vi "ma_Check Block Size (2ch) no State.vi"(0 "time signal X":waveform(dbl), 1 "averaging parameters":T3={"averaging mode"=enum."No averaging", "weighting mode"=enum."Exponential", "number of averages"=10} {"number of averages" min=1}, 5 "time signal Y":waveform(dbl), 9 "restart averaging (F)":bool, 11 "error in":errorcluster, 12 "caller VI name":string, 13 "state info":T1 {"Syy" format="%0.2f"; "Sxy" format="%0.2f"; "Sy" format="%0.2f"; "Sxx" format="%0.2f"; "avgs completed" format="%0.2f"; "df" format="%0.2f"; "Sx" format="%0.2f"; "spectrum parameters"."window" items=["Rectangle"=0, "Hanning"=1, "Hamming"=2, "Blackman-Harris"=3, "Exact Blackman"=4, "Blackman"=5, "Flat Top"=6, "4 Term B-Harris "=7, "7 Term B-Harris"=8, "Low Sidelobe"=9, "Blackman Nuttall"=11, "Triangle"=30, "Bartlett-Hanning"=31, "Bohman"=32, "Parzen"=33, "Welch"=34, "Kaiser"=60, "Dolph-Chebyshev"=61, "Gaussian"=62]; "dt" format="%0.2f"; "timestamp" format="%0.2f"; "dt history" format="%0.2f"; "t0 history" format="%0.2f"}) -> (4 "force restart averaging":bool, 14 "state info out":T1 {"Syy" format="%0.2f"; "Sxy" format="%0.2f"; "Sy" format="%0.2f"; "Sxx" format="%0.2f"; "avgs completed" format="%0.2f"; "df" format="%0.2f"; "Sx" format="%0.2f"; "spectrum parameters"."window" items=["Rectangle"=0, "Hanning"=1, "Hamming"=2, "Blackman-Harris"=3, "Exact Blackman"=4, "Blackman"=5, "Flat Top"=6, "4 Term B-Harris "=7, "7 Term B-Harris"=8, "Low Sidelobe"=9, "Blackman Nuttall"=11, "Triangle"=30, "Bartlett-Hanning"=31, "Bohman"=32, "Parzen"=33, "Welch"=34, "Kaiser"=60, "Dolph-Chebyshev"=61, "Gaussian"=62]; "dt" format="%0.2f"; "timestamp" format="%0.2f"; "dt history" format="%0.2f"; "t0 history" format="%0.2f"}, 15 "error out":errorcluster)   [LabVIEW 2020, in "NI_MAPro.lvlib"]
uses:
  NI_MAPro.lvlib
  2-chan State.ctl
  windowTd.ctl
  NI_MABase.lvlib
  NI_AALPro.lvlib
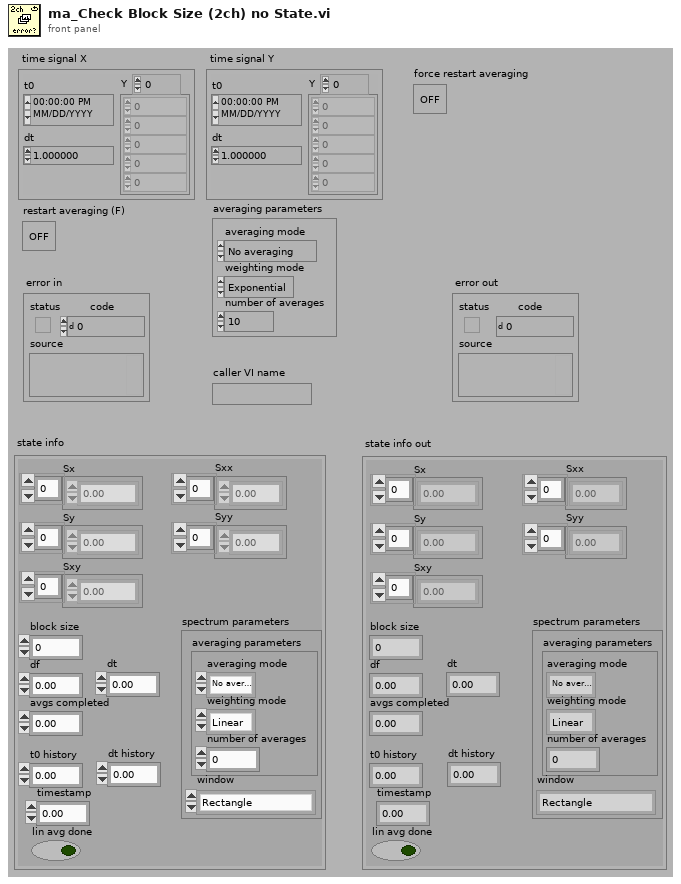
[diagram p1: front panel]
types:
  T1 = typedef "NI_MAPro.lvlib/2-chan State.ctl" = cluster{"Sx":cdb[], "Sy":cdb[], "Sxx":dbl[], "Syy":dbl[], "Sxy":cdb[], "block size":i32, "df":dbl, "dt":dbl, "avgs completed":dbl, "spectrum parameters":cluster{"averaging parameters":cluster{"averaging mode":enum16{"No averaging", "Vector averaging", "RMS averaging", "Peak hold"}, "weighting mode":enum16{"Linear", "Exponential"}, "number of averages":u32}, "window":T2}, "lin avg done":bool, "t0 history":dbl, "dt history":dbl, "timestamp":dbl}
  T2 = typedef "NI_AALPro.lvlib/windowTd.ctl" = u32
  T3 = cluster{"averaging mode":enum16{"No averaging", "Vector averaging", "RMS averaging", "Peak hold"}, "weighting mode":enum16{"Linear", "Exponential"}, "number of averages":u32}
  T4 = enum16{"No averaging", "Vector averaging", "RMS averaging", "Peak hold"}
  T5 = cluster{"status":bool, "code":i32, "caller VI name":string}
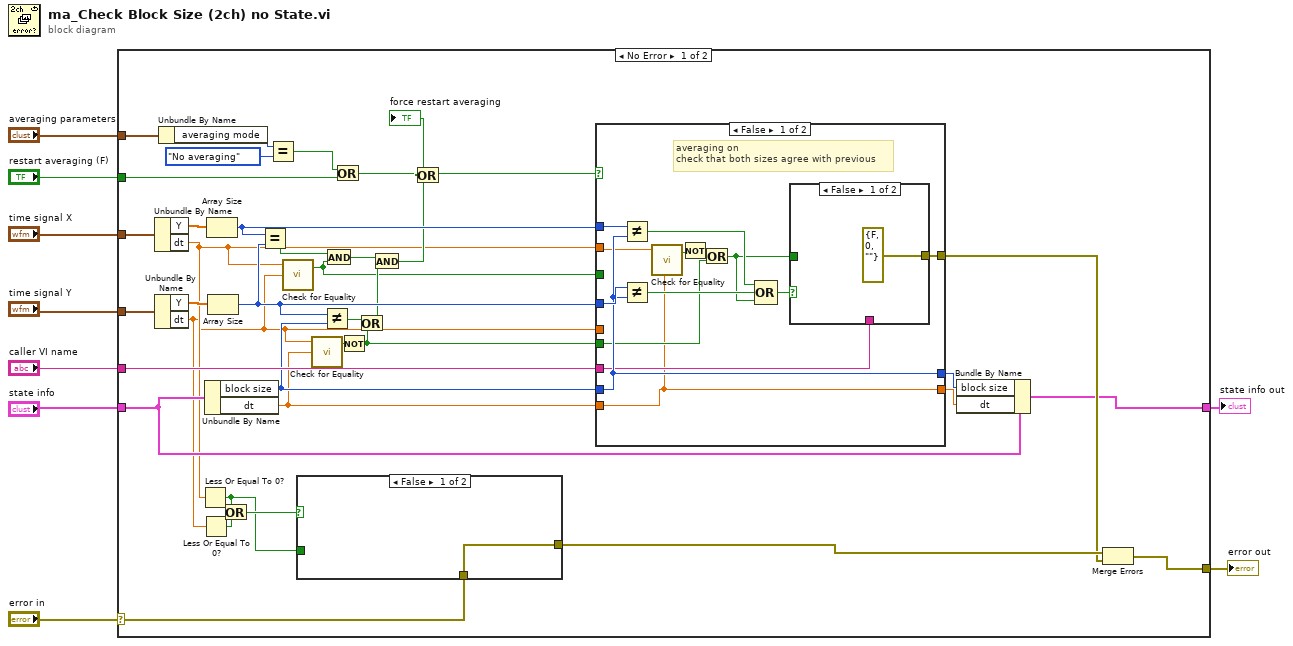
[diagram p0: block diagram]
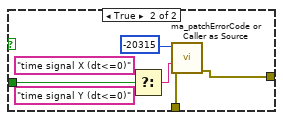
[diagram p2: hidden frame]
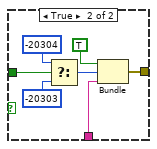
[diagram p3: hidden frame]
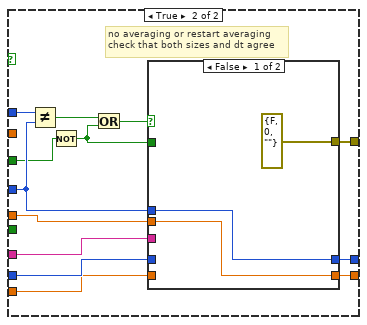
[diagram p4: hidden frame]
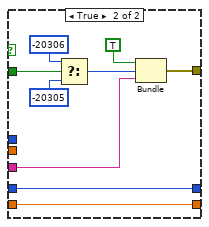
[diagram p5: hidden frame]
diagram:
  n1 = case shown="No Error" "error in" {
    selector: "error in" -> [w10 w103]
    tunnel: [w39 w103] -> w9
    tunnel: "time signal Y" -> [w46 _]
    tunnel: "time signal X" -> [w45 _]
    tunnel: "restart averaging (F)" -> [w44 _]
    tunnel: "averaging parameters" -> [w43 _]
    tunnel: "caller VI name" -> [w42 _]
    tunnel: "state info" -> [w38 w102]
    tunnel: [w17 w102] -> w1
    frame No Error {
      n2 = Unbundle By Name(w45) -> ("Y"=w37:dbl[], "dt"=w16:dbl)
      n3 = Unbundle By Name(w46) -> ("Y"=w36:dbl[], "dt"=w15:dbl)
      n4 = Unbundle By Name(w43) -> ("averaging mode"=w34:T4)
      n5 = Less Or Equal To 0?(x=w16) -> (x <= 0?=w21:bool)
      n6 = Less Or Equal To 0?(x=w15) -> (x <= 0?=w22:bool)
      n7 = Unbundle By Name(w38) -> ("block size"=w20:i32, "dt"=w14:dbl)
      n8 = Array Size(array=w37) -> (size(s)=w32:i32)
      n9 = Array Size(array=w36) -> (size(s)=w30:i32)
      n10 = Or(x=w21, y=w22) -> (x .or. y?=w23:bool)
      n11 = Equal?(x=w32, y=w30) -> (x = y?=w31:bool)
      n12 = Equal?(x=w34, y=T4."No averaging" ("averaging mode")) -> (x = y?=w33:bool)
      n13 = call "Check for Equality.vi"("n2"=w15, "n1"=w16) -> ("equal?"=w12:bool)  [unwired: 1 in, 1 out]
      n14 = case shown="False" w23 {
        tunnel: [w47 w49] -> w41
        tunnel: w21 -> [_ w52]
        tunnel: w10 -> [w47 w48]
        frame False {
        }
        frame True {
          n15 = Select(t="time signal X (dt<=0)", s=w52, f="time signal Y (dt<=0)") -> (s? t:f=w50:string)
          n16 = call "ma_patchErrorCode or Caller as Source.vi"("error in (no error)"=w48, "string to append to source"=w50, "error code"=-20315 ("code")) -> ("error out"=w49:errorcluster)  [unwired: 1 in, 7 out]
        }
      }
      n17 = call "Check for Equality.vi"("n2"=w14, "n1"=w15) -> ("equal?"=w13:bool)  [unwired: 1 in, 1 out]
      n18 = Not Equal?(x=w30, y=w20) -> (x != y?=w29:bool)
      n19 = And(x=w31, y=w12) -> (x .and. y?=w28:bool)
      n20 = Or(x=w33, y=w44) -> (x .or. y?=w25:bool)
      n21 = Not(x=w13) -> (.not. x?=w11:bool)
      n22 = Or(x=w29, y=w11) -> (x .or. y?=w27:bool)
      n23 = And(x=w28, y=w27) -> (x .and. y?=w24:bool)
      "force restart averaging" <- w24
      n24 = Or(x=w25, y=w24) -> (x .or. y?=w26:bool)
      n25 = case shown="False" w26 {
        tunnel: w32 -> [w68 w89]
        tunnel: w16 -> [w57 _]
        tunnel: w30 -> [w67 w86]
        tunnel: w15 -> [_ w84]
        tunnel: w20 -> [w65 w83]
        tunnel: w14 -> [w56 w82]
        tunnel: [w65 w87] -> w19
        tunnel: [w56 w85] -> w18
        tunnel: w42 -> [w60 w79]
        tunnel: [w63 w78] -> w40
        tunnel: w12 -> [_ w77]
        tunnel: w11 -> [w59 _]
        frame False {
          # "averaging on\ncheck that both sizes agree with previous"
          n26 = Not Equal?(x=w68, y=w65) -> (x != y?=w66:bool)
          n27 = Not Equal?(x=w67, y=w65) -> (x != y?=w64:bool)
          n28 = call "Check for Equality.vi"("n2"=w56, "n1"=w57) -> ("equal?"=w58:bool)  [unwired: 1 in, 1 out]
          n29 = Not(x=w58) -> (.not. x?=w55:bool)
          n30 = Or(x=w55, y=w59) -> (x .or. y?=w62:bool)
          n31 = Compound Arithmetic op=OR(w66, w64, w62) -> (w61:bool)
          n32 = case shown="False" w61 {
            tunnel: [errorcluster {"status"=FALSE, "code"=0, "source"=""} ("error in") w72] -> w63
            tunnel: w62 -> [_ w71]
            tunnel: w60 -> [_ w70]
            frame False {
            }
            frame True {
              n33 = Select(t=-20304 ("code"), s=w71, f=-20303 ("code")) -> (s? t:f=w74:i32)
              n34 = Bundle("status"=TRUE, "code"=w74, "caller VI name"=w70) -> (w72:T5)  [unwired: 1 out]
            }
          }
        }
        frame True {
          # "no averaging or restart averaging\ncheck that both sizes and dt agree"
          n35 = Not Equal?(x=w89, y=w86) -> (x != y?=w88:bool)
          n36 = Not(x=w77) -> (.not. x?=w80:bool)
          n37 = Or(x=w88, y=w80) -> (x .or. y?=w81:bool)
          n38 = case shown="False" w81 {
            tunnel: [w92 w101] -> w87
            tunnel: w86 -> [w92 _]
            tunnel: [w91 w100] -> w85
            tunnel: w84 -> [w91 _]
            tunnel: w83 -> [_ w101]
            tunnel: w82 -> [_ w100]
            tunnel: w80 -> [_ w99]
            tunnel: [errorcluster {"status"=FALSE, "code"=0, "source"=""} ("error in") w94] -> w78
            tunnel: w79 -> [_ w93]
            frame False {
            }
            frame True {
              n39 = Select(t=-20306 ("code"), s=w99, f=-20305 ("code")) -> (s? t:f=w95:i32)
              n40 = Bundle("status"=TRUE, "code"=w95, "caller VI name"=w93) -> (w94:T5)  [unwired: 1 out]
            }
          }
        }
      }
      n41 = Bundle By Name(cluster=w38, "block size"=w19, "dt"=w18) -> (w17:T1)
      n42 = Merge Errors(w41, w40) -> (w39:errorcluster)
    }
    frame Error {
    }
  }
  "error out" <- w9
  "state info out" <- w1
